vi "message_dio_control.vi"(11 "usermessage":string) -> ()   [LabVIEW 2012]
uses:
  <vilib>/eio/EIONode/EIONode.xnode
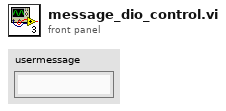
[diagram p1: front panel]
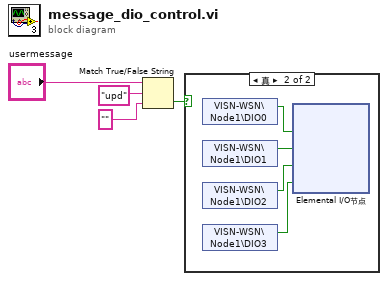
[diagram p0: block diagram]
diagram:
  n1 = Match True/False String(2:"" ("假字符串"), 3:"upd" ("真字符串"), 4:"usermessage") -> (0:w2:bool)  [unwired: 1 out]
  n2 = case shown="真" w2 {
    frame False {
    }
    frame True {
      n3 = shared-variable "VISN-WSN\\Node1\\DIO0"() -> (w8:bool)  [unwired: 1 in, 1 out]
      n4 = shared-variable "VISN-WSN\\Node1\\DIO1"() -> (w7:bool)  [unwired: 1 in, 1 out]
      n5 = shared-variable "VISN-WSN\\Node1\\DIO2"() -> (w6:bool)  [unwired: 1 in, 1 out]
      n6 = shared-variable "VISN-WSN\\Node1\\DIO3"() -> (w5:bool)  [unwired: 1 in, 1 out]
      n7 = xnode "Elemental I/O节点"("DIO0"=w8, "DIO1"=w7, "DIO2"=w6, "DIO3"=w5) -> ()  [unwired: 4 in, 4 out]
    }
  }
